vi "create_new.vi"(6 "Optional":T1, 9 "Labels":string[](array[string]), 10 "Properties":map{string, string}(c390)) -> (3 "New Target":refnum<class "target.lvclass">)   [LabVIEW 2020, in "datasources.lvlib" / "target.lvclass"]
uses:
  target.lvclass
  dataset/dataset.lvclass
  nominal types/channelConfig/channelConfig.lvclass
  target.lvclass/target.ctl
  properties.set.vi
  labels.set.vi
  dataset.set.vi
  channelConfig.set.vi
  nominal types/labels/labels.lvclass
  nominal types/properties/properties.lvclass
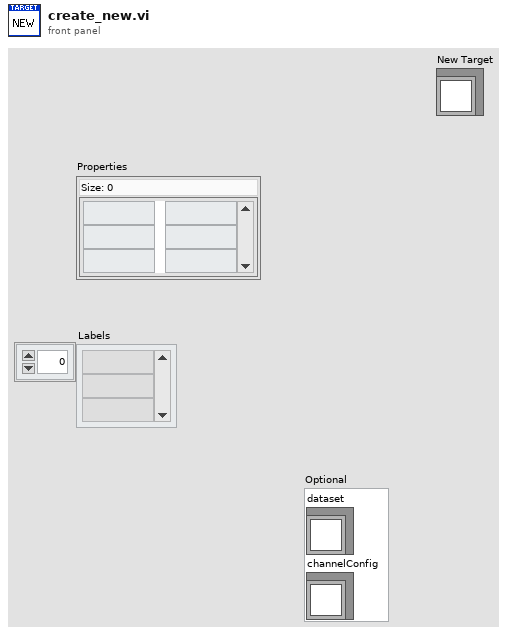
[diagram p1: front panel]
types:
  T1 = cluster{"dataset":refnum<class "dataset.lvclass">, "channelConfig":refnum<class "channelConfig.lvclass">}
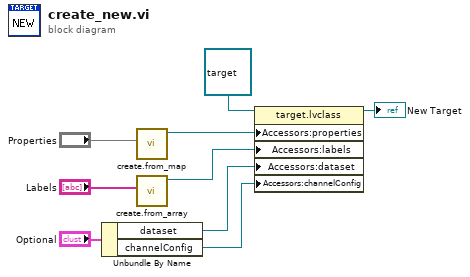
[diagram p0: block diagram]
diagram:
  n1 = Unbundle By Name("Optional") -> ("dataset"=w7:refnum<class "dataset.lvclass">, "channelConfig"=w6:refnum<class "channelConfig.lvclass">)
  n2 = call "create.from_map.vi"("properties"="Properties") -> ("properties out"=w2:refnum<class "properties.lvclass">)  [unwired: 9 in, 1 out]
  n3 = call "create.from_array.vi"("labels"="Labels") -> ("labels out"=w4:refnum<class "labels.lvclass">)  [unwired: 9 in, 1 out]
  n4 = property class="target.lvclass"(reference=refnum<class "target.lvclass"> refnum ("Target"), "Accessors:properties"=w2, "Accessors:labels"=w4, "Accessors:dataset"=w7, "Accessors:channelConfig"=w6) -> (reference out=→"New Target":refnum<class "target.lvclass">)  [unwired: 1 in, 1 out]
